vi "nanocal -- nuclear schottky goodness -- for UCO -- V3.vi"(3 "output control":T1, 4 "data":variant, 5 "X":dbl[](array[numeric])) -> (0 "error out":errorcluster, 1 "gradient":dbl[](array[numeric]), 2 "f(X)":dbl)   [LabVIEW 2020]
doc: "This template is the starting point for creating an objectivel function to be passed to the Unconstrained Optimization.vi."
uses:
  publisher action.ctl
  nanocal-goodness-weighting-strategy.ctl
  3-lorentzian-heat-response -- analytic derivatives V3.vi
  array -- integrate scalar product.vi
  array -- 3-finitediff.vi
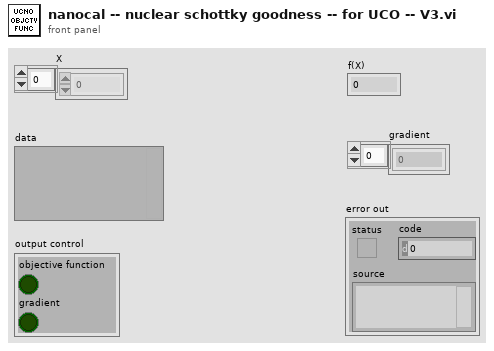
[diagram p1: front panel]
types:
  T1 = cluster{"objective function":bool, "gradient":bool}
  T2 = typedef "nanocal-goodness-weighting-strategy.ctl" = enum16{"as is", "|dz/dω|", "ω", "phase"}
  T3 = typedef "publisher action.ctl" = enum16{"set", "get", "init", "check"}
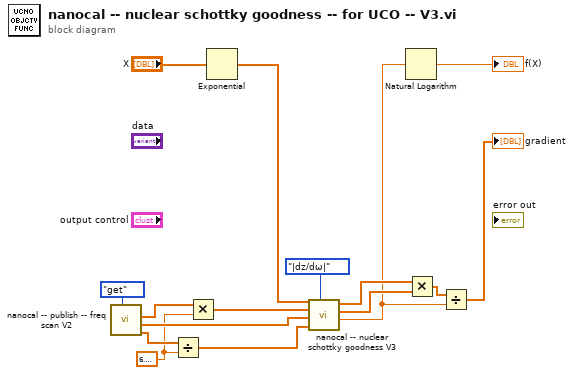
[diagram p0: block diagram]
diagram:
  w10 = 6.283185307179586
  n1 = call "nanocal -- publish -- freq scan V2.vi"("publisher action"=publisher_action."get") -> ("dz/dω out (V)"=w11:cdb[], "z out (V)"=w13:cdb[], "ω out (Hz)"=w15:dbl[])  [unwired: 8 in]
  n2 = Divide(x=w11, y=w10) -> (x/y=w12:cdb[])
  n3 = Multiply(x=w15, y=w10) -> (x*y=w14:dbl[])
  n4 = Exponential(1:"X") -> (0:w3:dbl[])
  n5 = call "nanocal -- nuclear schottky goodness V3.vi"("weighting strategy"=nanocal-goodness-weighting-strategy."|dz/dω|", "dz/dω IN (V)"=w12, "Voltage IN (V)"=w13, "ω (rad/sec)"=w14, "parameters"=w3) -> ("G"=w2:dbl, "derivatives"=w6:dbl[], "parameters OUT"=w9:dbl[])  [unwired: 2 in, 2 out]
  n6 = Natural Logarithm(1:w2) -> (0:→"f(X)":dbl)
  n7 = Multiply(x=w9, y=w6) -> (x*y=w8:dbl[])
  n8 = Divide(x=w8, y=w2) -> (x/y=→"gradient":dbl[])
